vi "Interpolate Y (single).vi"(8 "error in (no error)":errorcluster, 10 "x (0)":dbl, 11 "XY-data":cluster{"X-array":dbl[], "Y-array":dbl[]}) -> (0 "error out":errorcluster, 2 "y":dbl, 3 "XY-data out":cluster{"X-array":dbl[], "Y-array":dbl[]} {"Y-array" format="%.2p"; "X-array" format="%.2p"})   [LabVIEW 2019, in "xy_utilities.lvlib"]
doc: "Shift the zero value of the x array by giving a new fractional x index.\n\nWire data to the data input to determine the polymorphic instance to use or manually select the instance."
uses:
  xy_utilities.lvlib
  Sort (single).vi
  <userlib>/_OpenG.lib/array/array.llb/Sort Array__ogtk.vi
  <userlib>/_OpenG.lib/array/array.llb/Sort 1D Array (DBL)__ogtk.vi
  <userlib>/_OpenG.lib/array/array.llb/Reorder Array2__ogtk.vi
  <userlib>/_OpenG.lib/array/array.llb/Reorder 1D Array2 (DBL)__ogtk.vi
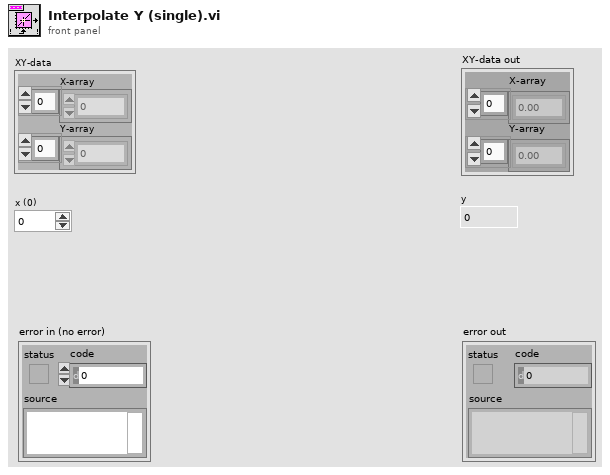
[diagram p1: front panel]
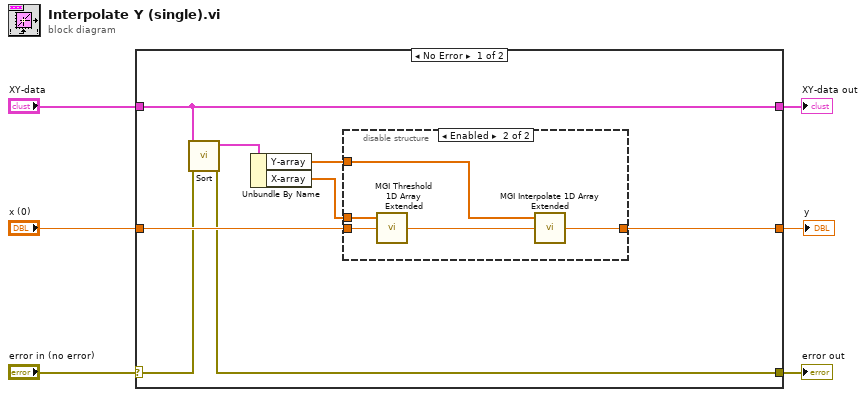
[diagram p0: block diagram]
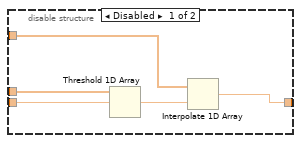
[diagram p2: hidden frame]
diagram:
  n1 = case shown="No Error" "error in (no error)" {
    selector: "error in (no error)" -> [w10 w26]
    tunnel: [w9 w26] -> w5
    tunnel: "XY-data" -> [w7 w25]
    tunnel: [w7 w25] -> w3
    tunnel: "x (0)" -> [w13 _]
    tunnel: [w14 _] -> w1
    frame No Error {
      n2 = call-poly "Sort.vi"("error in (no error)"=w10, "XY-data"=w7) -> ("error out"=w9:errorcluster, "Sorted XY-data out"=w8:cluster{"X-array":dbl[], "Y-array":dbl[]})  [unwired: 7 in, 1 out]
      n3 = Unbundle By Name(w8) -> ("Y-array"=w12:dbl[], "X-array"=w11:dbl[])
      n4 = disable-structure shown="Enabled" {
        disable-tunnel: [w19 w20] -> w14
        disable-tunnel: w13 -> [w17 w22]
        disable-tunnel: w12 -> [w15 w21]
        disable-tunnel: w11 -> [w16 w23]
        frame Disabled {
          n5 = Threshold 1D Array(2:w17, 3:w16) -> (0:w18:dbl)  [unwired: 1 in]
          n6 = Interpolate 1D Array(1:w18, 2:w15) -> (0:w19:dbl)
        }
        frame Enabled {
          n7 = call <userlib>:"MGI Threshold 1D Array Extended.vi"("Threshold Y"=w22, "Y Value[]"=w23) -> ("Extended Fractional Index"=w24:dbl)  [unwired: 1 in]
          n8 = call <userlib>:"MGI Interpolate 1D Array Extended.vi"("Fractional X"=w24, "Y Value[]"=w21) -> ("ExtendedY"=w20:dbl)  [unwired: 1 in]
        }
      }
    }
    frame Error {
    }
  }
  "error out" <- w5
  "XY-data out" <- w3
  "y" <- w1
